vi "comparison.vi"() -> ()   [LabVIEW 2019]
panel:
  in  "stop":bool
  out "c":dbl
  in  "b":dbl
  in  "a":dbl
  out "Numeric":i32
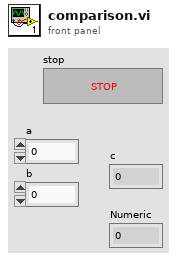
[diagram p1: front panel]
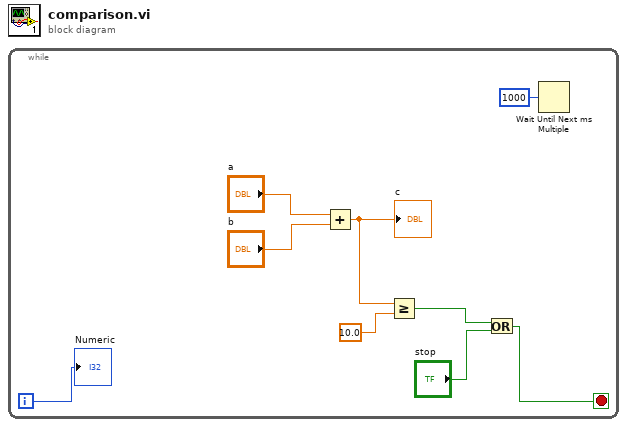
[diagram p0: block diagram]
diagram:
  n1 = while {
    i -> [w9]
    stop <- w2 stop-if-true
    n2 = Add(x="a", y="b") -> (x+y=w5:dbl)
    "c" <- w5
    n3 = Greater Or Equal?(x=w5, y=10.0) -> (x >= y?=w3:bool)
    n4 = Or(x=w3, y="stop") -> (x .or. y?=w2:bool)
    n5 = Wait Until Next ms Multiple(millisecond multiple=u32 1000) -> ()  [unwired: 1 out]
    "Numeric" <- w9
  }
